vi "DMA.Consolidate Transfers.vi"(8 "error in (no error)":errorcluster, 10 "DMA Transfers":T1[](array[typedef]) {"Block Descriptors"."next descriptor ptr" format="%08x"; "Block Descriptors"."data size" format="%08x"; "Block Descriptors"."data ptr (upper)" format="%08x"; "Block Descriptors"."data ptr (lower)" format="%08x"; "Block Descriptors"."descriptor ptr (aligned)" format="%08x"; "Block Descriptors"."descriptor size" format="%08x"; "Block Descriptors"."descriptor ptr (VISA)" format="%08x"; "RFM Address" format="%08x"}, 11 "GE 5565PIORC in":refnum<class "GE 5565PIORC Old.lvclass">) -> (0 "error out":errorcluster, 2 "Consolidated DMA Transfers":T1[](array[typedef]) {"Block Descriptors"."next descriptor ptr" format="%08x"; "Block Descriptors"."data size" format="%08x"; "Block Descriptors"."data ptr (upper)" format="%08x"; "Block Descriptors"."data ptr (lower)" format="%08x"; "Block Descriptors"."descriptor ptr (aligned)" format="%08x"; "Block Descriptors"."descriptor size" format="%08x"; "Block Descriptors"."descriptor ptr (VISA)" format="%08x"; "RFM Address" format="%08x"}, 3 "GE 5565PIORC out":refnum<class "GE 5565PIORC Old.lvclass">)   [LabVIEW 2016, in "GE 5565PIORC Old.lvclass"]
uses:
  GE 5565PIORC Old.lvclass
  Controls/DMA Transfer Spec.ctl
  Controls/DMA Block Descriptor.ctl
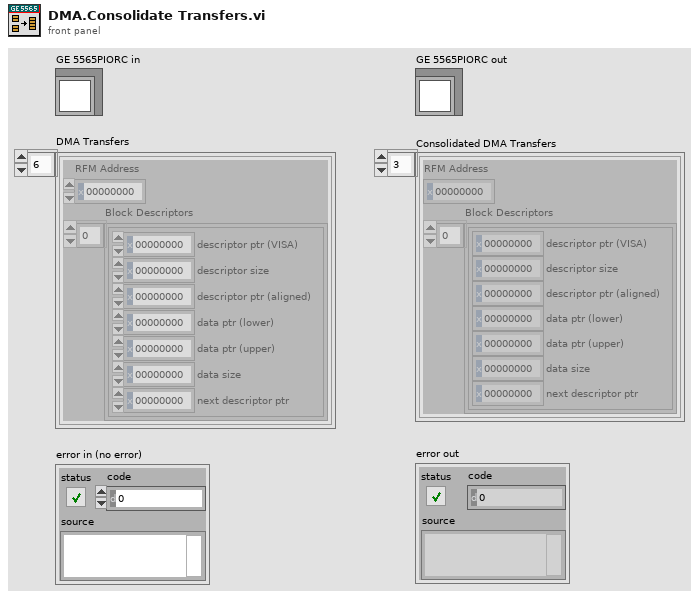
[diagram p1: front panel]
types:
  T1 = typedef "GE 5565PIORC Old.lvclass/DMA Transfer Spec.ctl" = cluster{"RFM Address":u32, "Block Descriptors":T2[]}
  T2 = typedef "GE 5565PIORC Old.lvclass/DMA Block Descriptor.ctl" = cluster{"descriptor ptr (VISA)":u32, "descriptor size":u32, "descriptor ptr (aligned)":u32, "data ptr (lower)":u32, "data ptr (upper)":u32, "data size":u32, "next descriptor ptr":u32}
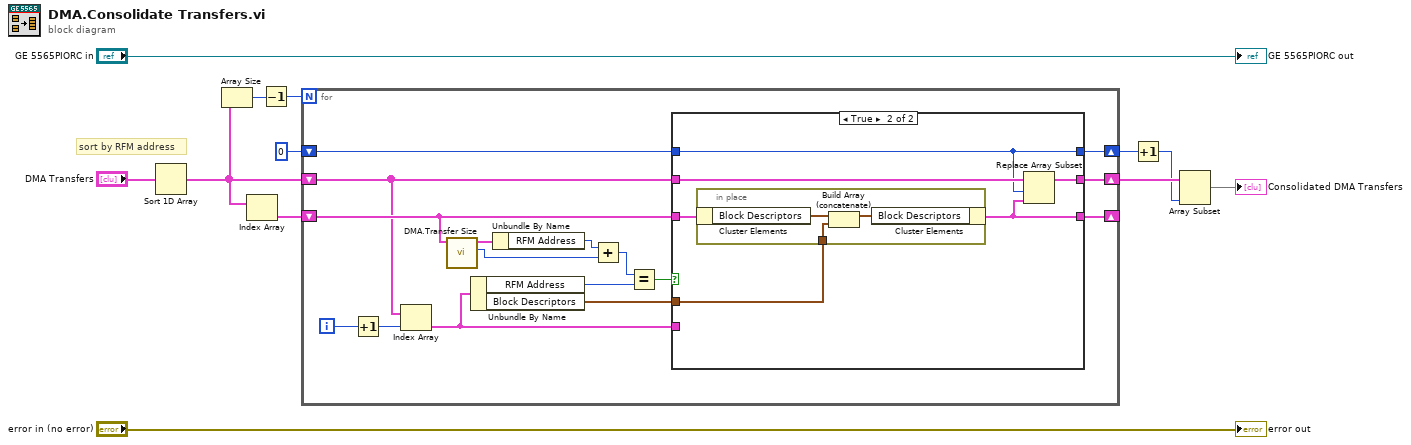
[diagram p0: block diagram]
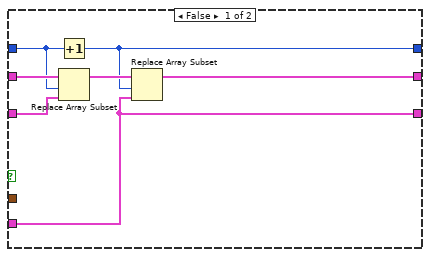
[diagram p2: hidden frame]
diagram:
  # "sort by RFM address"
  n1 = Sort 1D Array(array="DMA Transfers") -> (sorted array=w5:T1[])
  n2 = Array Size(array=w5) -> (size(s)=w9:i32)
  n3 = Index Array(array=w5) -> (element=w6:T1)  [unwired: 1 in]
  n4 = Decrement(x=w9) -> (x-1=w8:i32)
  n5 = for {
    N: w8 -> [_]
    shift-right: [w16] -> w3
    shift-left: w5 -> [w13]
    shift-right: [w17] -> w4
    shift-left: 0 -> [w14]
    shift-right: [w18] -> _
    shift-left: w6 -> [w15]
    i -> [w20]
    n6 = Increment(x=w20) -> (x+1=w28:i32)
    n7 = Index Array(array=w13, index=w28) -> (element=w19:T1)
    n8 = call "DMA.Transfer Size.vi"("DMA Transfer Spec"=w15) -> ("Transfer Size (bytes)"=w25:u32, "DMA Transfer Spec out"=w27:T1)  [unwired: 9 in]
    n9 = Unbundle By Name(w19) -> ("RFM Address"=w23:u32, "Block Descriptors"=w21:T2[])
    n10 = Unbundle By Name(w27) -> ("RFM Address"=w26:u32)
    n11 = Add(x=w26, y=w25) -> (x+y=w24:u32)
    n12 = Equal?(x=w24, y=w23) -> (x = y?=w22:bool)
    n13 = case shown="True" w22 {
      tunnel: w13 -> [w35 w39]
      tunnel: w21 -> [_ w40]
      tunnel: w15 -> [w34 w41]
      tunnel: w14 -> [w33 w37]
      tunnel: [w29 w38] -> w16
      tunnel: [w31 w36] -> w18
      tunnel: [w30 w37] -> w17
      tunnel: w19 -> [w31 _]
      frame False {
        n14 = Increment(x=w33) -> (x+1=w30:i32)
        n15 = Replace Array Subset(array=w35, new element=w34, index=w33) -> (w32:T1[])
        n16 = Replace Array Subset(array=w32, new element=w31, index=w30) -> (w29:T1[])
      }
      frame True {
        n17 = in-place {
          in-place-border: w40 -> [w42]
          n18 = in-place-cluster #1(w41) -> ("Block Descriptors"=w44:T2[])
          n19 = Build Array (concatenate)(w44, w42) -> (w43:T2[])
          n20 = in-place-cluster #1("Block Descriptors"=w43) -> (w36:T1)
        }
        n21 = Replace Array Subset(array=w39, new element=w36, index=w37) -> (w38:T1[])
      }
    }
  }
  n22 = Increment(x=w4) -> (x+1=w2:i32)
  n23 = Array Subset(array=w3, length=w2) -> (→"Consolidated DMA Transfers":T1[])  [unwired: 1 in]
  "error out" <- "error in (no error)"
  "GE 5565PIORC out" <- "GE 5565PIORC in"
